vi "SAC-Compute ASTF.vi"(0 "speaker path":path, 1 "Window":T1, 11 "Error In":errorcluster, 12 "Desired Fs":dbl) -> (15 "error out":errorcluster)   [LabVIEW 2020]
uses:
  HRTF VIs/Typedefs/HRTF-Window.ctl
  HRTF VIs/Typedefs/HRTF-Window Type.ctl
  HRTF VIs/Typedefs/HRTF-filt Cluster.ctl
  Type Defs/Cal Stimulus.ctl
  <vilib>/Analysis/2dsp.llb/Real FFT.vi
  <vilib>/Analysis/2dsp.llb/Inverse Real FFT.vi
  <vilib>/Analysis/baseanly.llb/Mean.vi
  <vilib>/Analysis/baseanly.llb/Mean (DBL).vi
  Utility VIs/Math VIs/dB to Linear (scalar).vi
  <vilib>/Analysis/2dsp.llb/Rational Resample (single channel, DBL).vi
  Utility VIs/Math VIs/FFT x(t) to dB,Degrees (1D).vi
  <userlib>/_matio/level5/Public/Write/Append Data Element.llb/Append Data Element (Anything).vi
  <vilib>/Analysis/NI_AALPro.lvlib
  <userlib>/_matio/level5.lvlib
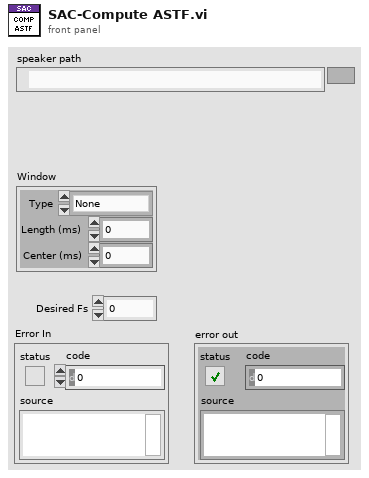
[diagram p1: front panel]
types:
  T1 = typedef "HRTF-Window.ctl" = cluster{"Type":T2, "Length (ms)":dbl, "Center (ms)":dbl}
  T2 = typedef "HRTF-Window Type.ctl" = enum16{"None", "Rectangle", "Hanning"}
  T3 = typedef "Cal Stimulus.ctl" = cluster{"Min Freq (Hz)":dbl, "Max Freq (Hz)":dbl, "Freq Step (Hz)":dbl, "Waveform":enum16{"Chirp", "Weighted"}, "Attenuation (dB)":dbl, "Sample Rate (Hz)":dbl}
  T4 = enum16{"big-endian, network order", "native, host order", "little-endian"}
  T5 = typedef "HRTF-filt Cluster.ctl" = cluster{"Type":string, "Fs":dbl, "a":dbl[], "b":dbl[], "window":i32, "Length_ms":dbl, "Center_ms":dbl}
  T6 = typedef "SAC-Parameters.ctl" = cluster{"Fs (Hz)":dbl, "atten (dB)":dbl, "Waveform":T7, "Freq Res (Hz)":dbl, "Order":i32, "Averages":i32, "seed":i64, "Window":T1, "Mic gain":dbl, "Mic sens":dbl}
  T7 = typedef "HRTF-Waveform.ctl" = enum16{"Chirp", "MLS"}
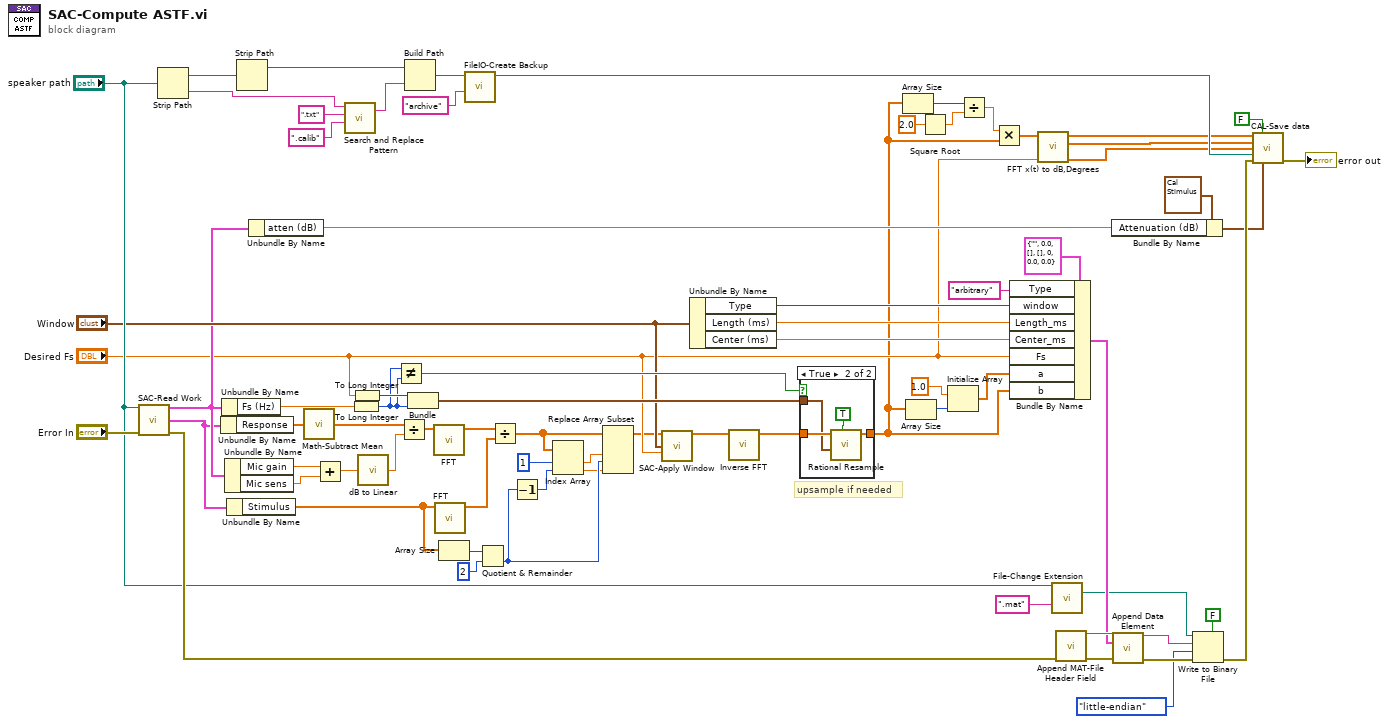
[diagram p0: block diagram]
diagram:
  # "upsample if needed"
  n1 = call "SAC-Read Work.vi"("path"="speaker path", "Error In"="Error In") -> ("Params"=w27:T6, "Result"=w25:cluster{"Stimulus":dbl[], "Response":dbl[]}, "error out"=w45:errorcluster)  [unwired: 11 in]
  n2 = Strip Path(path="speaker path") -> (stripped path=w62:path, name=w61:string)
  n3 = Unbundle By Name(w25) -> ("Response"=w41:dbl[])
  n4 = Unbundle By Name(w27) -> ("Fs (Hz)"=w49:dbl)
  n5 = Unbundle By Name(w27) -> ("Mic gain"=w32:dbl, "Mic sens"=w31:dbl)
  n6 = Unbundle By Name(w25) -> ("Stimulus"=w4:dbl[])
  n7 = Strip Path(path=w62) -> (stripped path=w58:path)  [unwired: 1 out]
  n8 = Unbundle By Name(w27) -> ("atten (dB)"=w26:dbl)
  n9 = call "Math-Subtract Mean.vi"("Y"=w41) -> ("Y - mean(Y)"=w12:dbl[])  [unwired: 4 in]
  n10 = Add(x=w32, y=w31) -> (x+y=w30:dbl)
  n11 = call <vilib>:"Search and Replace Pattern.vi"("string"=w61, "regular expression (\"\")"=".txt" ("regular expression (\"\")"), "replace string (\"\")"=".calib" ("replace string (\"\")")) -> ("result string"=w57:string)  [unwired: 2 in, 1 out]
  n12 = To Long Integer(number=w49) -> (32bit integer=w47:i32)
  n13 = To Long Integer(number="Desired Fs") -> (32bit integer=w50:i32)
  n14 = call-poly "dB to Linear.vi"("dB"=w30) -> ("linear"=w28:dbl)
  n15 = Not Equal?(x=w47, y=w47) -> (x != y?=w46:bool)
  n16 = Divide(x=w12, y=w28) -> (x/y=w29:dbl[])
  n17 = Build Path(base path=w58, name or relative path=w57) -> (appended path=w56:path)
  n18 = Bundle(w50, w47) -> (w48:cluster{i32, i32})  [unwired: 1 in]
  n19 = call-poly <vilib>:"FFT.vi"("X"=w29) -> ("FFT {X}"=w33:cdb[])  [unwired: 9 in, 1 out]
  n20 = call-poly <vilib>:"FFT.vi"("X"=w4) -> ("FFT {X}"=w10:cdb[])  [unwired: 9 in, 1 out]
  n21 = Array Size(array=w4) -> (size(s)=w9:i32)
  n22 = call "FileIO-Create Backup.vi"("Subfolder"="archive", "Path"=w56) -> ("Path (thru)"=w40:path)  [unwired: 6 in, 3 out]
  n23 = Quotient & Remainder(x=w9, y=2) -> (floor(x/y)=w3:i32)  [unwired: 1 out]
  n24 = Divide(x=w33, y=w10) -> (x/y=w7:cdb[])
  n25 = Decrement(x=w3) -> (x-1=w2:i32)
  n26 = Index Array(array=w7, index #1=1 ("index"), index #2=w2) -> (element #1=w5:cdb, element #2=w1:cdb)
  n27 = Replace Array Subset(array=w7, new element #1=w5, new element #2=w1, index #2=w3) -> (w11:cdb[])  [unwired: 1 in]
  n28 = call "SAC-Apply Window.vi"("Array in"=w11, "Window"="Window", "Fs (Hz)"="Desired Fs") -> ("Array out"=w24:cdb[])  [unwired: 12 in]
  n29 = Unbundle By Name("Window") -> ("Type"=w53:T2, "Length (ms)"=w52:dbl, "Center (ms)"=w51:dbl)
  n30 = call-poly <vilib>:"Inverse FFT.vi"("FFT {X}"=w24) -> ("X"=w34:dbl[])  [unwired: 9 in, 1 out]
  n31 = case shown="True" w46 {
    tunnel: w34 -> [w75 w79]
    tunnel: [w75 w78] -> w21
    tunnel: w48 -> [_ w77]
    frame False {
    }
    frame True {
      n32 = call-poly <vilib>:"Rational Resample.vi"("reset"=TRUE, "resample factor"=w77, "X"=w79) -> ("Y"=w78:dbl[])  [unwired: 6 in, 2 out]
    }
  }
  n33 = Array Size(array=w21) -> (size(s)=w20:i32)
  n34 = Array Size(array=w21) -> (size(s)=w71:i32)
  n35 = Square Root(x=2.0) -> (sqrt(x)=w17:dbl)
  n36 = Initialize Array(1.0 ("element"), w71) -> (w72:dbl[])
  n37 = Divide(x=w20, y=w17) -> (x/y=w19:dbl)
  n38 = Multiply(x=w19, y=w21) -> (x*y=w22:dbl[])
  n39 = Bundle By Name(cluster=T5 {"Type"="", "Fs"=0.0, "a"=[], "b"=[], "window"=0, "Length_ms"=0.0, "Center_ms"=0.0} ("filt"), "Type"="arbitrary", "window"=w53, "Length_ms"=w52, "Center_ms"=w51, "Fs"="Desired Fs", "a"=w72, "b"=w21) -> (w67:T5)
  n40 = call-poly "FFT x(t) to dB,Degrees.vi"("Fs (Hz)"="Desired Fs", "X"=w22) -> ("Freq (Hz)"=w14:dbl[], "+Freq Phase of FFT (degrees)"=w15:dbl[], "+Freq. Mag of FFT (dB rms)"=w16:dbl[])  [unwired: 7 in]
  n41 = call "File-Change Extension.vi"("Path"="speaker path", "new extension"=".mat" ("replace string (\"\")")) -> ("new path"=w42:path)  [unwired: 13 in]
  n42 = call <userlib>:"Append MAT-File Header Field.vi"("error"=w45) -> ("result string"=w68:string, "error out"=w69:errorcluster)  [unwired: 13 in]
  n43 = Bundle By Name(cluster=T3 {"Min Freq (Hz)"=50.0, "Max Freq (Hz)"=50000.0, "Freq Step (Hz)"=50.0, "Waveform"=enum."Chirp", "Attenuation (dB)"=20.0, "Sample Rate (Hz)"=100000.0} ("Cal Stimulus"), "Attenuation (dB)"=w26) -> (w35:T3)
  n44 = call-poly <userlib>:"Append Data Element.vi"("initial string"=w68, "data"=w67, "error in (no error)"=w69) -> ("result string"=w65:string, "error out"=w66:errorcluster)  [unwired: 11 in]
  n45 = Write to Binary File(file (use dialog)=w42, data=w65, error in=w66, 5:FALSE ("prepend array or string size? (T)"), 9:T4."little-endian" ("byte order (0:big-endian, network order)")) -> (error out=w39:errorcluster)  [unwired: 1 in, 2 out]
  n46 = call "CAL-Save data.vi"("Mag"=w16, "backup"=FALSE, "Phase"=w15, "Frequency"=w14, "path"=w40, "error in (no error)"=w39, "Cal Stimulus"=w35) -> ("error out"=→"error out":errorcluster)  [unwired: 7 in, 1 out]
